vi "VLine1006.vi"   [LabVIEW 2013]
uses:
  <vilib>/Heliosphere Research LLC/Advanced Plotting Toolkit/api_annotations/HVLineProperties.ctl
  <vilib>/Heliosphere Research LLC/Advanced Plotting Toolkit/properties/Line.ctl
  <vilib>/Heliosphere Research LLC/Advanced Plotting Toolkit/properties/Line_Style.ctl
  <vilib>/Heliosphere Research LLC/Advanced Plotting Toolkit/typedefs/PlotColor.ctl
  <vilib>/Heliosphere Research LLC/Advanced Plotting Toolkit/properties/Display.ctl
  <vilib>/Heliosphere Research LLC/Advanced Plotting Toolkit/api_annotations/TextProperties.ctl
  <vilib>/Heliosphere Research LLC/Advanced Plotting Toolkit/properties/Text.ctl
  <vilib>/Heliosphere Research LLC/Advanced Plotting Toolkit/properties/Text_FontSize.ctl
  <vilib>/Heliosphere Research LLC/Advanced Plotting Toolkit/properties/Text_FontStyle.ctl
  <vilib>/Heliosphere Research LLC/Advanced Plotting Toolkit/Advanced Plotting Toolkit.lvlib
types:
  T1 = typedef "Advanced Plotting Toolkit.lvlib/Text_FontSize.ctl" = i32
  T2 = typedef "Advanced Plotting Toolkit.lvlib/TextProperties.ctl" = cluster{"Text":T3, "Display":T6}
  T3 = typedef "Advanced Plotting Toolkit.lvlib/Text.ctl" = cluster{"Color":T4, "Background Color":T4, "Font Size (points)":T1, "Font Style":T5, "Rotation Angle":dbl}
  T4 = typedef "Advanced Plotting Toolkit.lvlib/PlotColor.ctl" = u32
  T5 = typedef "Advanced Plotting Toolkit.lvlib/Text_FontStyle.ctl" = enum16{"Automatic", "Normal", "Italic", "Bold"}
  T6 = typedef "Advanced Plotting Toolkit.lvlib/Display.ctl" = cluster{"Alpha":dbl, "Z Order":dbl}
  T7 = typedef "Advanced Plotting Toolkit.lvlib/HVLineProperties.ctl" = cluster{"Line":T8, "Display":T6}
  T8 = typedef "Advanced Plotting Toolkit.lvlib/Line.ctl" = cluster{"Style":T9, "Color":T4, "Width":sgl}
  T9 = typedef "Advanced Plotting Toolkit.lvlib/Line_Style.ctl" = enum16{"Automatic", "Solid", "Dashed", "Dotted", "Dash-dot", "Invisible"}
  T10 = typedef "Advanced Plotting Toolkit.lvlib/PlotID.ctl" = i32
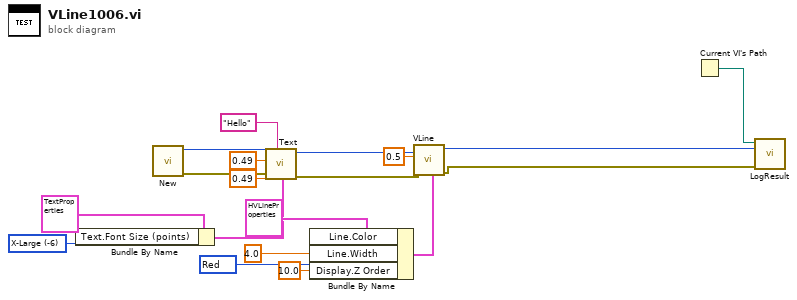
[diagram p0: block diagram]
diagram:
  w2 = T1 -6 items=["Automatic"=0, "XX-Small"=-1, "X-Small"=-2, "Small"=-3, "Medium"=-4, "Large"=-5, "X-Large"=-6, "XX-Large"=-7] ("Text.Font Size (points)")
  w12 = T4 16711680 items=["Automatic"=2147483647, "Black"=0, "White"=16777215, "Red"=16711680, "Green"=2263842, "Blue"=255, "Cyan"=65535, "Magenta"=16711935, "Yellow"=16776960] ("Line.Color")
  n1 = Bundle By Name(cluster=T2 {"Text"={"Color"=2147483647, "Background Color"=2147483647, "Font Size (points)"=0, "Font Style"=enum."Automatic", "Rotation Angle"=nan}, "Display"={"Alpha"=nan, "Z Order"=nan}} ("Text Properties"), "Text.Font Size (points)"=w2) -> (w3:T2)
  n2 = call <vilib>:"New.vi"() -> ("error out"=w9:errorcluster, "Plot ID"=w11:T10)  [unwired: 10 in]
  n3 = call <vilib>:"Text.vi"("Properties"=w3, "Text"="Hello", "error in (no error)"=w9, "Y Position"=0.49, "X Position"=0.49, "Plot ID"=w11) -> ("error out"=w8:errorcluster, "Plot ID Out"=w10:T10)  [unwired: 4 in]
  n4 = Bundle By Name(cluster=T7 {"Line"={"Style"=enum."Automatic", "Color"=2147483647, "Width"=nan}, "Display"={"Alpha"=nan, "Z Order"=nan}} ("Axis Line Properties"), "Line.Color"=w12, "Line.Width"=sgl 4.0, "Display.Z Order"=10.0) -> (w14:T7)
  n5 = call <vilib>:"VLine.vi"("Properties"=w14, "error in (no error)"=w8, "X (data coords)"=0.5 ("Y (data coords)"), "Plot ID"=w10) -> ("error out"=w16:errorcluster, "Plot ID Out"=w17:T10)  [unwired: 6 in]
  n6 = Current VI's Path() -> (path=w19:path)
  n7 = call "LogResult.vi"("Test Result"=w16, "Test Artifact"=w17, "VI Path"=w19) -> ()  [unwired: 9 in]
